vi "Autonomous 1 Container.vi"(11 "Cluster":T1) -> ()   [LabVIEW 2014]
uses:
  Autonomous 1 Container States.ctl
  <vilib>/Rock Robotics/WPI/RobotDrive/WPI_RobotDriveGetSetRefNum.vi
  <vilib>/Rock Robotics/WPI/RobotDrive/WPI_RobotDriveArcadeDrive_Standard(NoSaturation).vi
panel:
  in  "Detect Platform":bool
  in  "Wheel Encoder":dbl
  in  "Back Arm Encoder":dbl
  out "Lift Back arms":bool
  out "Move forward":bool
  out "Move parallel to SP":bool
  out "Stop once at Autozone":bool
  out "Close Back arms":bool
  out "Start":bool
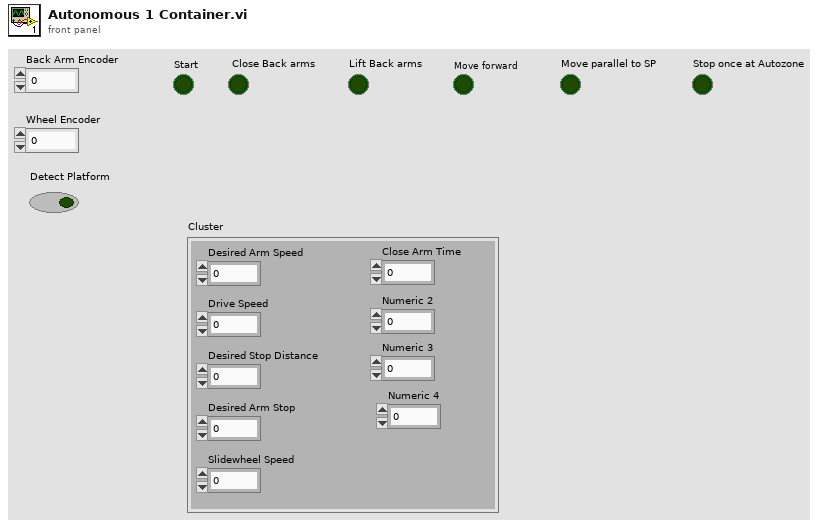
[diagram p1: front panel]
types:
  T1 = cluster{"Desired Arm Speed":dbl, "Drive Speed":dbl, "Desired Stop Distance":dbl, "Desired Arm Stop":dbl, "Slidewheel Speed":dbl, "Close Arm Time":dbl, "Numeric 2":dbl, "Numeric 3":dbl, "Numeric 4":dbl}
  T2 = typedef "Autonomous 1 Container States.ctl" = enum16{"Start", "Close Back Arms", "Lift back arms", "Move forward ", "Move parallel left to scoring plat", "Stop once at autozone"}
  T3 = typedef "WPI_MotorControlDeviceRef.ctl" = cluster{"DeviceStatus":errorcluster, "Type":T4, "PWM":cluster{"Controller":T5, "PWM Channel":T6, "DeadBand":T7}, "CAN":cluster{"Device Number":u8, "Control Mode":T8, "Semaphore":T9, "Max Vout":dbl, "TalonSRX Control Mode":T10}, "Invert":bool, "TransformRef":T11, "InvTransformRef":T11}
  T4 = typedef "WPI_MotorControlType.ctl" = enum16{"PWM", "CAN", "CANTalonSRX"}
  T5 = typedef "FPGA_TypedefDigitalModule.ctl" = enum16{"Controller 1"}
  T6 = typedef "FPGA_DIOPWMChannel.ctl" = enum8{"PWM 0", "PWM 1", "PWM 2", "PWM 3", "PWM 4", "PWM 5", "PWM 6", "PWM 7", "PWM 8", "PWM 9", "PWM MXP 0", "PWM MXP 1", "PWM MXP 2", "PWM MXP 3", "PWM MXP 4", "PWM MXP 5", "PWM MXP 6", "PWM MXP 7", "PWM MXP 8", "PWM MXP 9", "Invalid"}
  T7 = typedef "WPI_PWMDeadband.ctl" = cluster{"Name":string, "maxPositivePwm":i32, "minPositivePwm":i32, "centerPwm":i32, "maxNegativePwm":i32, "minNegativePwm":i32, "angularRange":u16}
  T8 = typedef "WPI_CANJaguar_ControlMode.ctl" = enum8{"Percent VBus", "Current", "Speed", "Position", "Voltage"}
  T9 = typedef "Semaphore RefNum" = refnum<k1>
  T10 = typedef "WPI_CANTalonSRX_APIControlMode.ctl" = enum8{"Percent VBus", "Speed", "Position", "Slave", "Unchanged / Invalid"}
  T11 = typedef "WPI_PWMTransform_ConPane.ctl" = refnum<vi>
  T12 = typedef "WPI_RobotDriveDevRef.ctl" = cluster{"DevStatus":errorcluster, "Motors[]":T3[], "Square Inputs":bool, "Max Output":dbl}
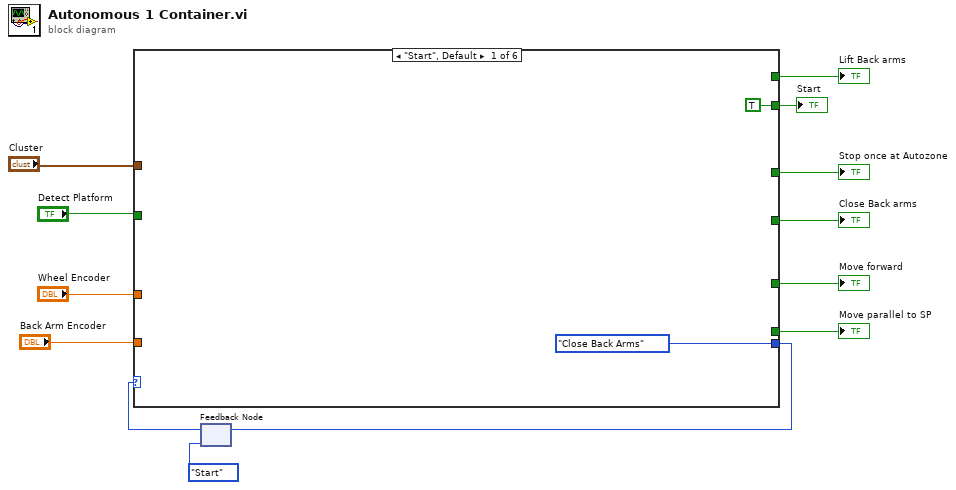
[diagram p0: block diagram]
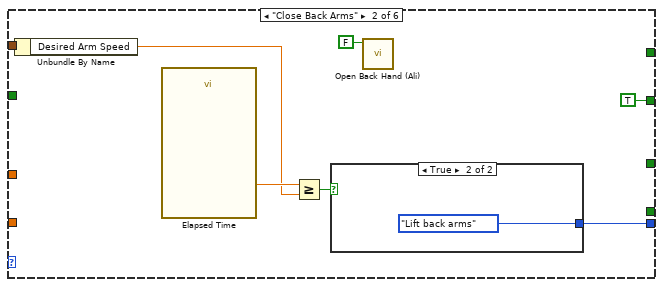
[diagram p2: hidden frame]
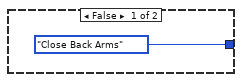
[diagram p3: hidden frame]
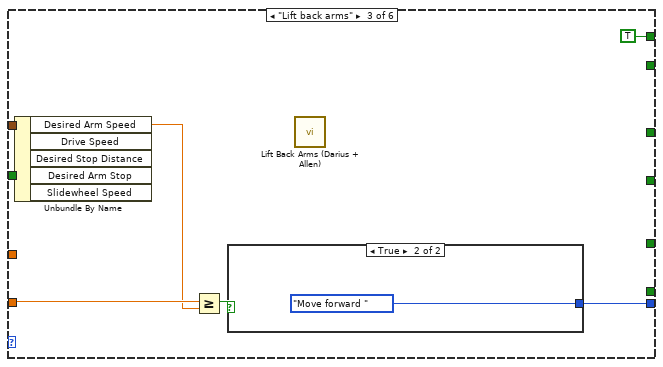
[diagram p4: hidden frame]
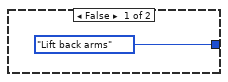
[diagram p5: hidden frame]
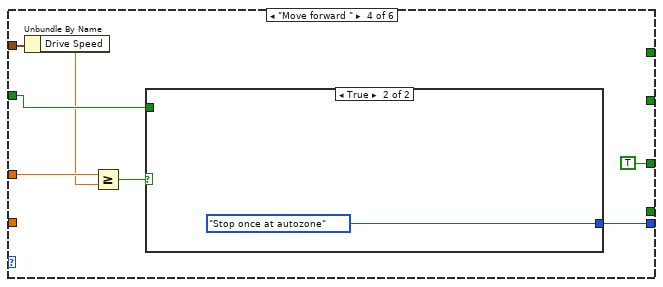
[diagram p6: hidden frame]
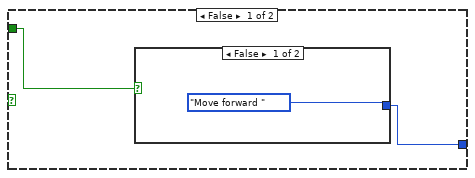
[diagram p7: hidden frame]
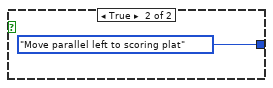
[diagram p8: hidden frame]
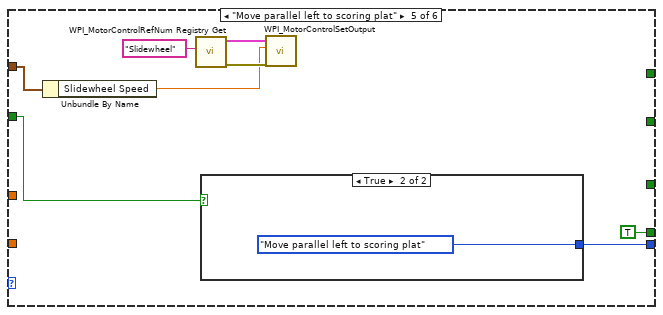
[diagram p9: hidden frame]
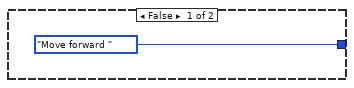
[diagram p10: hidden frame]
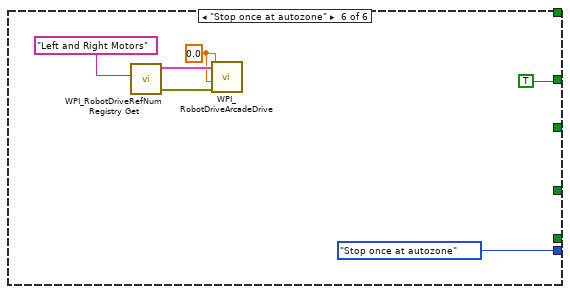
[diagram p11: hidden frame]
diagram:
  n1 = feedback #1(Autonomous_1_Container_States."Start") -> (w11:T2)
  n2 = case shown="\"Start\", Default" w11 {
    tunnel: [TRUE _ _ _ _ _] -> w12
    tunnel: [_ TRUE _ _ _ _] -> w10
    tunnel: [_ _ TRUE _ _ _] -> w9
    tunnel: [_ _ _ TRUE _ _] -> w8
    tunnel: [_ _ _ _ TRUE _] -> w7
    tunnel: [_ _ _ _ _ TRUE] -> w6
    tunnel: [Autonomous_1_Container_States."Close Back Arms" w19 w28 w38 w51 Autonomous_1_Container_States."Stop once at autozone"] -> w4
    tunnel: "Back Arm Encoder" -> [_ _ w29 _ _ _]
    tunnel: "Wheel Encoder" -> [_ _ _ w36 _ _]
    tunnel: "Detect Platform" -> [_ _ _ w35 w50 _]
    tunnel: "Cluster" -> [_ w17 w27 w34 w46 _]
    frame "Start", Default {
    }
    frame "Close Back Arms" {
      n3 = Unbundle By Name(w17) -> ("Desired Arm Speed"=w16:dbl)
      n4 = call "Elapsed Time"() -> ("Elapsed Time (s)"=w21:dbl)  [unwired: 12 in, 7 out]
      n5 = Greater Or Equal?(x=w21, y=w16) -> (x >= y?=w20:bool)
      n6 = case shown="True" w20 {
        tunnel: [Autonomous_1_Container_States."Close Back Arms" Autonomous_1_Container_States."Lift back arms"] -> w19
        frame False {
        }
        frame True {
        }
      }
      n7 = call "Open Back Hand (Ali).vi"("Open?"=FALSE) -> ()  [unwired: 11 in]
    }
    frame "Lift back arms" {
      n8 = Unbundle By Name(w27) -> ("Desired Arm Speed"=w26:dbl)  [unwired: 4 out]
      n9 = Greater Or Equal?(x=w29, y=w26) -> (x >= y?=w25:bool)
      n10 = case shown="True" w25 {
        tunnel: [Autonomous_1_Container_States."Lift back arms" Autonomous_1_Container_States."Move forward "] -> w28
        frame False {
        }
        frame True {
        }
      }
      n11 = call "Lift Back Arms (Darius + Allen).vi"() -> ()  [unwired: 12 in]
    }
    frame "Move forward " {
      n12 = Unbundle By Name(w34) -> ("Drive Speed"=w33:dbl)
      n13 = Greater Or Equal?(x=w36, y=w33) -> (x >= y?=w37:bool)
      n14 = case shown="True" w37 {
        tunnel: [w40 Autonomous_1_Container_States."Stop once at autozone"] -> w38
        tunnel: w35 -> [w41 _]
        frame False {
          n15 = case shown="False" w41 {
            tunnel: [Autonomous_1_Container_States."Move forward " Autonomous_1_Container_States."Move parallel left to scoring plat"] -> w40
            frame False {
            }
            frame True {
            }
          }
        }
        frame True {
        }
      }
    }
    frame "Move parallel left to scoring plat" {
      n16 = Unbundle By Name(w46) -> ("Slidewheel Speed"=w45:dbl)
      n17 = call <vilib>:"WPI_MotorControlRefNum Registry Get.vi"("refnum name"="Slidewheel") -> ("error out"=w47:errorcluster, "MotorControlDevRef"=w48:T3)  [unwired: 9 in]
      n18 = case shown="True" w50 {
        tunnel: [Autonomous_1_Container_States."Move forward " Autonomous_1_Container_States."Move parallel left to scoring plat"] -> w51
        frame False {
        }
        frame True {
        }
      }
      n19 = call <vilib>:"WPI_MotorControlSetOutput.vi"("error in (no error)"=w47, "Output"=w45, "MotorControlDevRef"=w48) -> ()  [unwired: 6 in, 3 out]
    }
    frame "Stop once at autozone" {
      w55 = 0.0 ("X axis value")
      n20 = call <vilib>:"WPI_RobotDriveRefNum Registry Get.vi"("refnum name"="Left and Right Motors") -> ("error out"=w56:errorcluster, "RobotDriveDevRef"=w57:T12)  [unwired: 1 in, 8 out]
      n21 = call-poly <vilib>:"WPI_RobotDriveArcadeDrive.vi"("error in (no error)"=w56, "Y axis value"=w55, "X axis value"=w55, "RobotDriveDevRef"=w57) -> ()  [unwired: 5 in, 3 out]
    }
  }
  "Start" <- w12
  "Close Back arms" <- w10
  "Stop once at Autozone" <- w6
  "Move parallel to SP" <- w7
  "Move forward" <- w8
  "Lift Back arms" <- w9
  n22 = feedback-in #1(w4) -> ()
